vi "SetCurrentTriple.vi"(8 "error in":errorcluster, 10 "Current":dbl[](array[numeric]), 11 "VISA resource name in":refnum<visa-resource-name>) -> (0 "error out":errorcluster, 3 "VISA resource name out":refnum<visa-resource-name>)   [LabVIEW 2012]
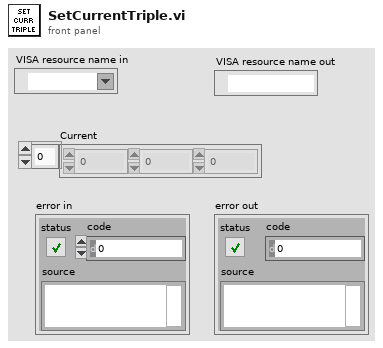
[diagram p1: front panel]
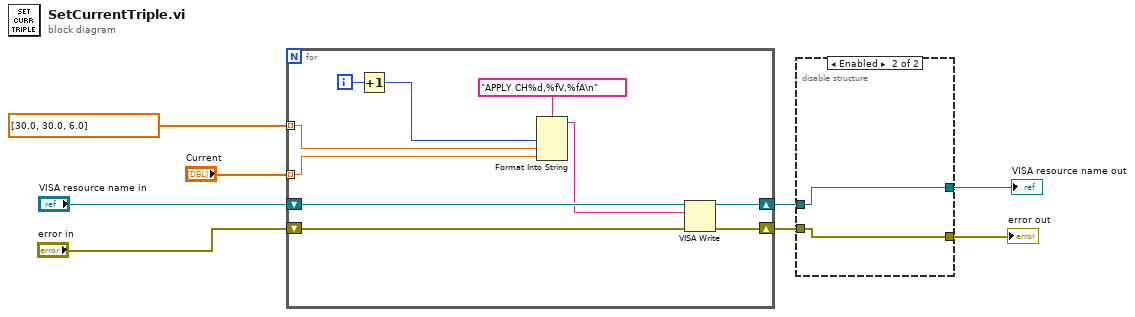
[diagram p0: block diagram]
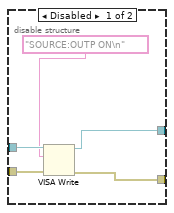
[diagram p2: hidden frame]
diagram:
  n1 = for {
    shift-right: [w18] -> w4
    shift-left: "VISA resource name in" -> [w16]
    shift-right: [w17] -> w2
    shift-left: "error in" -> [w15]
    tunnel: "Current" -> [w10] mode=indexing
    tunnel: dbl[] [30.0, 30.0, 6.0] -> [w11] mode=indexing
    i -> [w14]
    n2 = Increment(x=w14) -> (x+1=w12:i32)
    n3 = Format Into String(format string="APPLY CH%d,%fV,%fA\n", w12, w11, w10) -> (resulting string=w9:string)  [unwired: 2 in, 1 out]
    n4 = VISA Write(VISA resource name=w16, write buffer=w9, error in (no error)=w15) -> (VISA resource name out=w18:refnum<visa-resource-name>, error out=w17:errorcluster)  [unwired: 1 out]
  }
  n5 = disable-structure shown="Enabled" {
    disable-tunnel: w4 -> [w23 w25]
    disable-tunnel: [w22 w25] -> w3
    disable-tunnel: w2 -> [w21 w24]
    disable-tunnel: [w20 w24] -> w1
    frame Disabled {
      n6 = VISA Write(VISA resource name=w23, write buffer="SOURCE:OUTP ON\n", error in (no error)=w21) -> (VISA resource name out=w22:refnum<visa-resource-name>, error out=w20:errorcluster)  [unwired: 1 out]
    }
    frame Enabled {
    }
  }
  "VISA resource name out" <- w3
  "error out" <- w1
